vi "ClassNameCalcV2.vi"(6 "ClassName Cache":refnum<data-value>, 8 "error in (no error)":errorcluster, 9 "Deserialize":T7, 10 "wired object":refnum<class>, 11 "SerializedClassHeader (child,parent)":T5[](array[typedef])) -> (0 "error out":errorcluster, 2 "ClassOps (child, parent)":T1[](array[typedef]), 3 "Target Object":refnum<class "BlueSerializable.lvclass">)   [LabVIEW 2020, in "BlueSerialization.lvlib" / "BlueSerializer.lvclass"]
uses:
  BlueSerializer.lvclass
  DeserializeOptions.ctl
  DeserializeSlicingOptions.ctl
  DeserializeMutationOptions.ctl
  DeserializePreservationOptions.ctl
  PreserveNonWiredDataOption.ctl
  ClassHeader.ctl
  <vilib>/Utility/EditLVLibs/LibVersion.ctl
  ClassNameCacheMap.ctl
  ClassNameObj.ctl
  BlueSerializable/BlueSerializable.lvclass
  Support/SetSerializableDataClusterIterable.ctl
  Support/SetSerializableDataClusterLayer.ctl
  BlueSerializableVersion.ctl
  Support/SetSerializableDataObject.ctl
  <vilib>/Utility/error.llb/Clear Errors.vi
  <resource>/Framework/Providers/BlueSerializationProviderShared/GetVersionNumberFromMutation.vi
  <resource>/Framework/Providers/BlueSerializationProviderShared/FindMutationHistoryIndex.vi
  <resource>/Framework/Providers/BlueSerializationProviderShared/UserCommentToVersion.vi
  <vilib>/Utility/LVClass/Get LV Class Default Value By Name.vi
  <vilib>/Utility/error.llb/Error Cluster From Error Code.vi
  <vilib>/Utility/LVClass/Get LV Class Name.vi
  <vilib>/Utility/EditLVLibs/Edit LVLibs.lvlib
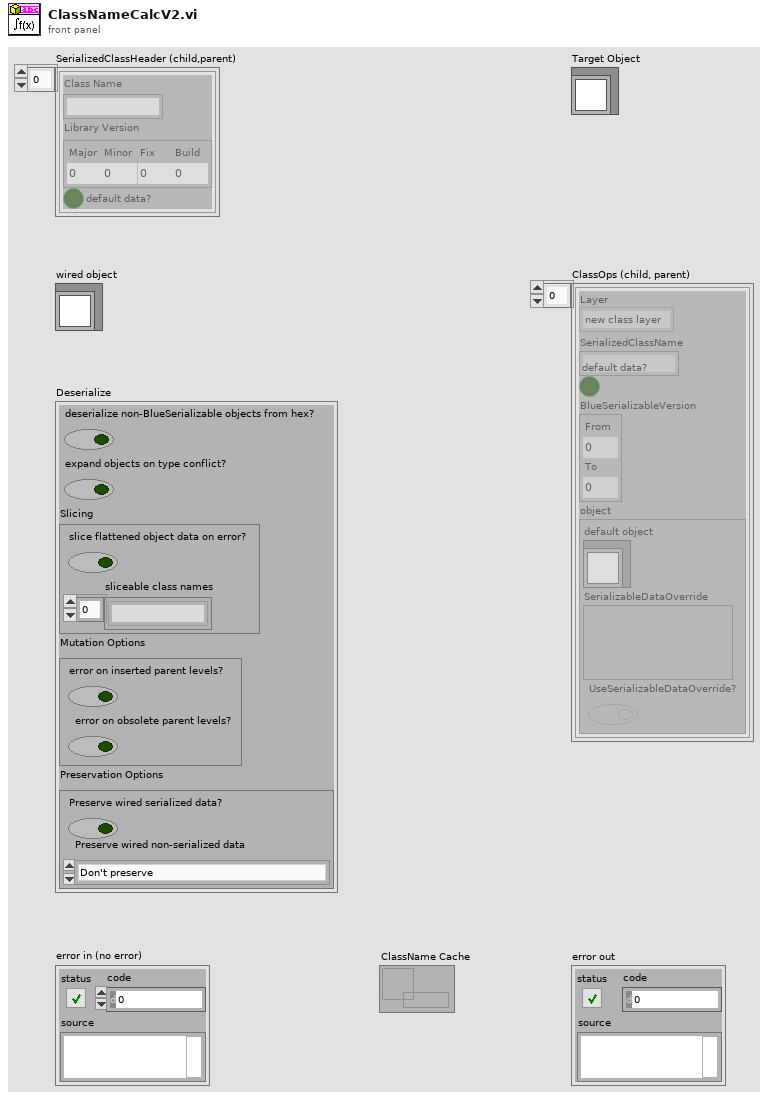
[diagram p1: front panel]
types:
  T1 = typedef "BlueSerialization.lvlib/BlueSerializer.lvclass/SetSerializableDataClusterIterable.ctl" = cluster{"Layer":T2, "SerializedClassName":string, "default data?":bool, "BlueSerializableVersion":T3, "object":T4}
  T2 = typedef "BlueSerialization.lvlib/BlueSerializer.lvclass/SetSerializableDataClusterLayer.ctl" = enum16{"new class layer", "dropped class layer", "agreed class layer"}
  T3 = typedef "BlueSerialization.lvlib/BlueSerializer.lvclass/BlueSerializableVersion.ctl" = cluster{"From":u16, "To":u16}
  T4 = typedef "BlueSerialization.lvlib/BlueSerializer.lvclass/SetSerializableDataObject.ctl" = cluster{"default object":refnum<class "BlueSerializable.lvclass">, "SerializableDataOverride":variant, "UseSerializableDataOverride?":bool}
  T5 = typedef "BlueSerialization.lvlib/BlueSerializer.lvclass/ClassHeader.ctl" = cluster{"Class Name":string, "Library Version":T6, "default data?":bool}
  T6 = typedef "Edit LVLibs.lvlib/LibVersion.ctl" = cluster{"Major":u16, "Minor":u16, "Fix":u16, "Build":u16}
  T7 = typedef "BlueSerialization.lvlib/BlueSerializer.lvclass/DeserializeOptions.ctl" = cluster{"deserialize non-BlueSerializable objects from hex?":bool, "expand objects on type conflict?":bool, "Slicing":T8, "Mutation Options":T9, "Preservation Options":T10}
  T8 = typedef "BlueSerialization.lvlib/BlueSerializer.lvclass/DeserializeSlicingOptions.ctl" = cluster{"slice flattened object data on error?":bool, "sliceable class names":string[]}
  T9 = typedef "BlueSerialization.lvlib/BlueSerializer.lvclass/DeserializeMutationOptions.ctl" = cluster{"error on inserted parent levels?":bool, "\terror on obsolete parent levels?":bool}
  T10 = typedef "BlueSerialization.lvlib/BlueSerializer.lvclass/DeserializePreservationOptions.ctl" = cluster{"Preserve wired serialized data?":bool, "Preserve wired non-serialized data":T11}
  T11 = typedef "BlueSerialization.lvlib/BlueSerializer.lvclass/PreserveNonWiredDataOption.ctl" = enum16{"Don't preserve", "Preserve (error on less-specific wired types)", "Preserve (except on less-specific wired types)"}
  T12 = typedef "Edit LVLibs.lvlib/Mutation History.ctl" = T13[]
  T13 = typedef "Edit LVLibs.lvlib/Mutation Record.ctl" = cluster{"Library Version":T6, "Old Name Index":u8, "Class Default Data":variant, "Cluster Order Map":u32[], "Parent Name":string, "Parent Path":path, "LabVIEW Version":u32, "User Comments":string, "Mutation Flags":u8, "Parent Old Name Index":u8, "Parent Levels Added":u16, "Parent Levels Removed":u16}
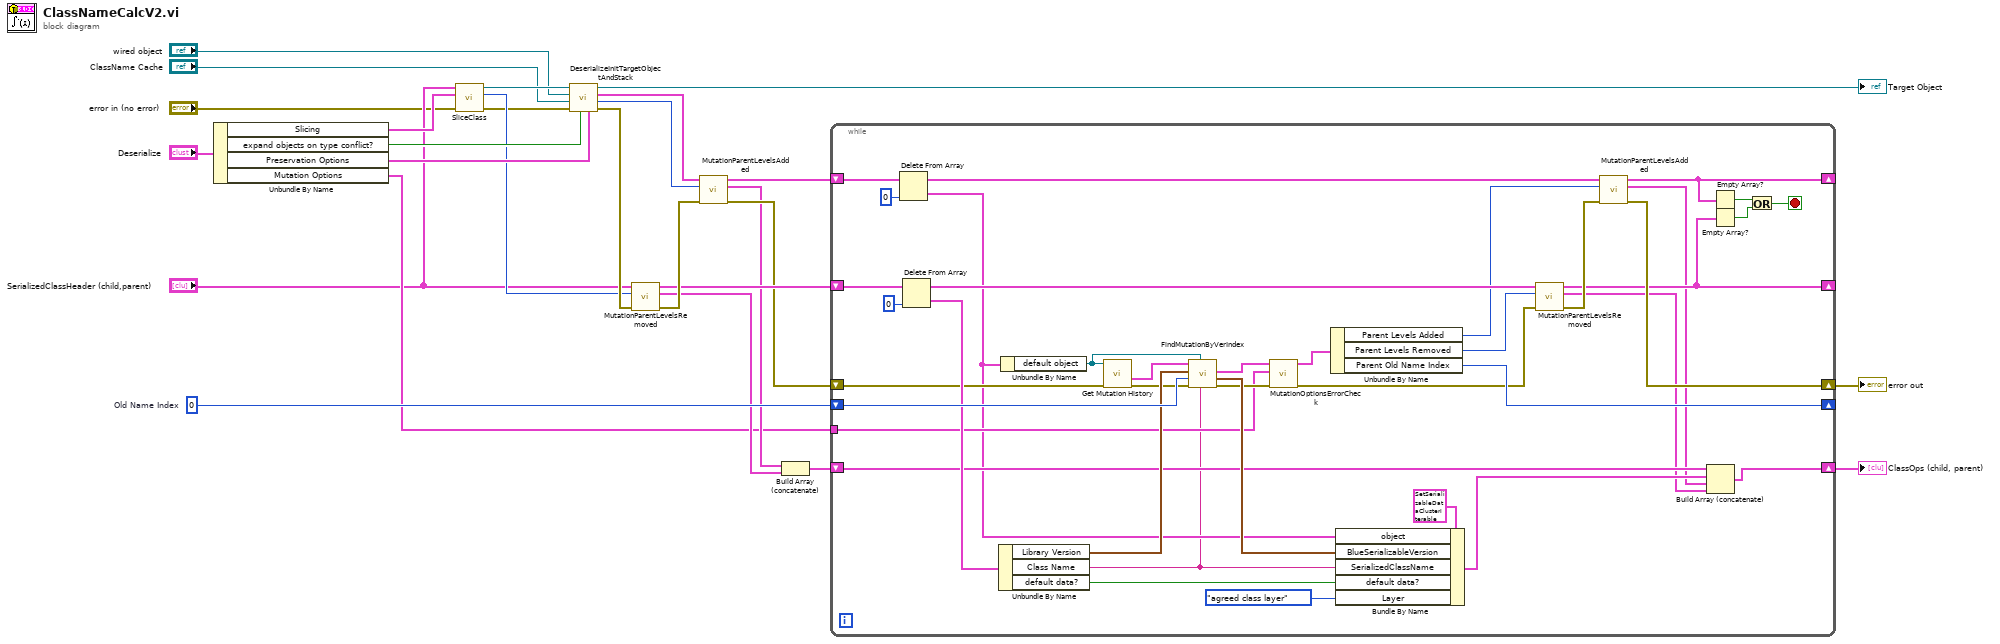
[diagram p0: block diagram]
diagram:
  w26 = u8 0  # Old Name Index
  n1 = Unbundle By Name("Deserialize") -> ("Slicing"=w12:T8, "expand objects on type conflict?"=w16:bool, "Preservation Options"=w15:T10, "Mutation Options"=w14:T9)
  n2 = call "SliceClass.vi"("error in (no error)"="error in (no error)", "Slicing"=w12, "SerializedClassHeader (child,parent)"="SerializedClassHeader (child,parent)") -> ("error IO"=w10:errorcluster, "NumLevelsSliced"=w11:u16, "from object (default value)"=w9:refnum<class>)  [unwired: 6 in]
  n3 = call "DeserializeInitTargetObjectAndStack.vi"("Preservation Options"=w15, "expand objects on type conflict?"=w16, "error in (no error)"=w10, "ClassName Cache"="ClassName Cache", "Wired object (not default)"="wired object", "From object (default value)"=w9) -> ("error out"=w17:errorcluster, "NumLevelsExpanded"=w13:u16, "Object stack (child, parent)"=w18:T4[], "Target Object"=→"Target Object":refnum<class "BlueSerializable.lvclass">)  [unwired: 2 in]
  n4 = call "MutationParentLevelsRemoved.vi"("error in (no error)"=w17, "Parent Levels Removed"=w11, "SerializedClassHeader (child,parent)"="SerializedClassHeader (child,parent)") -> ("error out"=w24:errorcluster, "ClassOps"=w20:T1[], "SerializedClassHeader (child,parent)"=w23:T5[])  [unwired: 6 in]
  n5 = call "MutationParentLevelsAdded.vi"("error in (no error)"=w24, "Parent Levels Added"=w13, "Object stack in (child, parent)"=w18) -> ("error out"=w22:errorcluster, "ClassOps"=w21:T1[], "Object stack out (child, parent)"=w25:T4[])  [unwired: 6 in]
  n6 = Build Array (concatenate)(w21, w20) -> (w19:T1[])
  n7 = while {
    shift-right: [w56] -> _
    shift-left: w26 -> [w64]
    shift-right: [w45] -> w1
    shift-left: w22 -> [w51]
    shift-right: [w44] -> _
    shift-left: w25 -> [w58]
    shift-right: [w43] -> _
    shift-left: w23 -> [w61]
    shift-right: [w38] -> w3
    shift-left: w19 -> [w39]
    tunnel: w14 -> [w31]
    stop <- w40 stop-if-true
    n8 = Delete From Array(array=w58, index=0) -> (deleted portion=w30:T4, array with subset deleted=w48:T4[])  [unwired: 1 in]
    n9 = Delete From Array(array=w61, index=0) -> (deleted portion=w55:T5, array with subset deleted=w50:T5[])  [unwired: 1 in]
    n10 = Unbundle By Name(w55) -> ("Library Version"=w54:T6, "Class Name"=w27:string, "default data?"=w29:bool)
    n11 = Unbundle By Name(w30) -> ("default object"=w28:refnum<class "BlueSerializable.lvclass">)
    n12 = call <vilib>:"Get Mutation History.vi"("error in"=w51, "Input object"=w28) -> ("error out"=w52:errorcluster, "Mutation History"=w65:T12)  [unwired: 6 in]
    n13 = call "FindMutationByVerIndex.vi"("SerializedClassName"=w27, "default object"=w28, "error in (no error)"=w52, "Old Name Index"=w64, "Library Version"=w54, "Mutation History"=w65) -> ("error out"=w35:errorcluster, "BlueSerializableVersion"=w63:T3, "Mutation Record"=w32:T13)  [unwired: 3 in]
    n14 = call "MutationOptionsErrorCheck.vi"("error in (no error)"=w35, "Mutation Options"=w31, "Mutation Record"=w32) -> ("error out"=w33:errorcluster, "Mutation Record"=w34:T13)  [unwired: 7 in]
    n15 = Unbundle By Name(w34) -> ("Parent Levels Added"=w47:u16, "Parent Levels Removed"=w49:u16, "Parent Old Name Index"=w56:u8)
    n16 = Bundle By Name(cluster=T1 {"Layer"=enum."new class layer", "SerializedClassName"="", "default data?"=FALSE, "BlueSerializableVersion"={"From"=0, "To"=0}, "object"={"default object"=refnum, "SerializableDataOverride"=variant(cluster{"SerializableData":variant, "Use?":bool} {"SerializableData"=variant, "Use?"=FALSE}), "UseSerializableDataOverride?"=FALSE}} ("Cluster 2"), "object"=w30, "BlueSerializableVersion"=w63, "SerializedClassName"=w27, "default data?"=w29, "Layer"=SetSerializableDataClusterLayer."agreed class layer") -> (w59:T1)
    n17 = call "MutationParentLevelsRemoved.vi"("error in (no error)"=w33, "Parent Levels Removed"=w49, "SerializedClassHeader (child,parent)"=w50) -> ("error out"=w46:errorcluster, "ClassOps"=w36:T1[], "SerializedClassHeader (child,parent)"=w43:T5[])  [unwired: 6 in]
    n18 = call "MutationParentLevelsAdded.vi"("error in (no error)"=w46, "Parent Levels Added"=w47, "Object stack in (child, parent)"=w48) -> ("error out"=w45:errorcluster, "ClassOps"=w37:T1[], "Object stack out (child, parent)"=w44:T4[])  [unwired: 6 in]
    n19 = Build Array (concatenate)(w39, w59, w37, w36) -> (w38:T1[])
    n20 = Empty Array?(array=w44) -> (empty?=w42:bool)
    n21 = Empty Array?(array=w43) -> (empty?=w41:bool)
    n22 = Or(x=w42, y=w41) -> (x .or. y?=w40:bool)
  }
  "error out" <- w1
  "ClassOps (child, parent)" <- w3
